vi "RT Errors.Write Numeric to Source (U64).vi"(9 "offset (0)":i32, 10 "value":u64, 11 "error in":errorcluster) -> (1 "new offset":i32, 3 "error out":errorcluster)   [LabVIEW 2016, in "RT Error Handling.lvlib"]
uses:
  RT Error Handling.lvlib
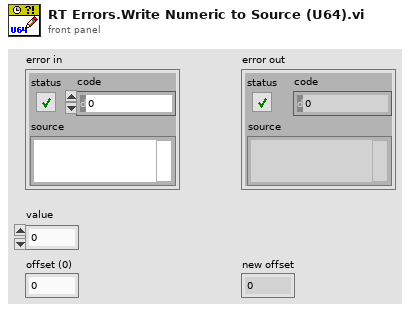
[diagram p1: front panel]
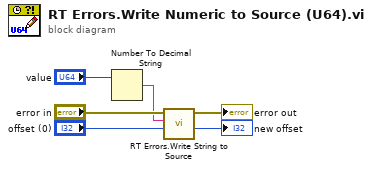
[diagram p0: block diagram]
diagram:
  n1 = Number To Decimal String(number="value") -> (decimal integer string=w1:string)  [unwired: 1 in]
  n2 = call "RT Errors.Write String to Source.vi"("offset (0)"="offset (0)", "string"=w1, "error in"="error in") -> ("new offset"=→"new offset":i32, "error out"=→"error out":errorcluster)  [unwired: 7 in]
